vi "Get visa 1d DBL data.vi"(7 "VISA resource name":refnum<visa-resource-name>, 8 "error in (no error)":errorcluster, 9 "Name":string, 10 "Mag Lab Parameters in":refnum<class "Mag Lab Parameters.lvclass">, 11 "HP counter in":refnum<class "HP counter.lvclass">) -> (0 "error out":errorcluster, 1 "Channel data":dbl[](array[numeric]), 2 "Channel names":string[](array[string]), 3 "HP counter out":refnum<class "HP counter.lvclass">, 5 "VISA resource name out":refnum<visa-resource-name>)   [LabVIEW 2015, in "HP counter.lvclass"]
uses:
  HP counter.lvclass
  Mag Lab Properties/Mag Lab Parameters.lvclass
  Counter/Counter Parameters.ctl
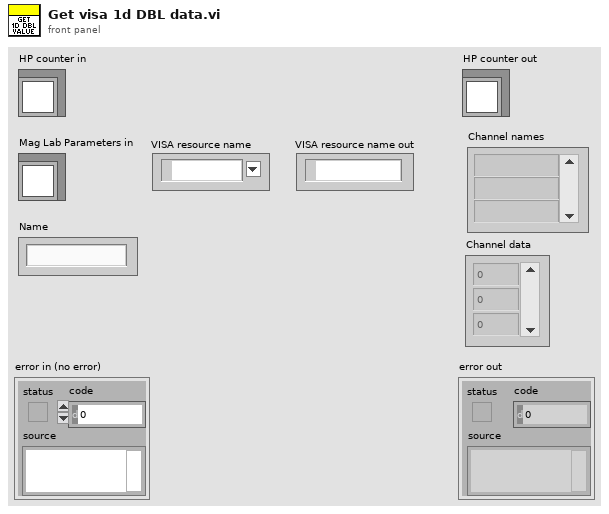
[diagram p1: front panel]
types:
  T1 = typedef "Counter Parameters.ctl" = cluster{"Channels to measure":i32[]}
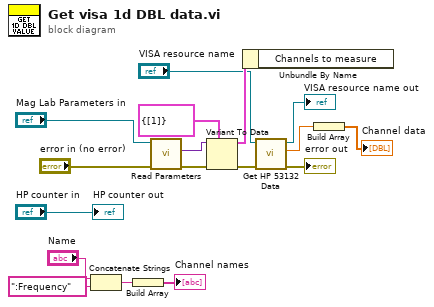
[diagram p0: block diagram]
diagram:
  n1 = Concatenate Strings("Name", ":Frequency" ("string")) -> (w7:string)
  n2 = Build Array(w7) -> (→"Channel names":string[])
  n3 = call-dynamic "Read Parameters.vi"("error in (no error)"="error in (no error)", "Mag Lab Parameters in"="Mag Lab Parameters in") -> ("error out"=w13:errorcluster, "Parameters"=w16:variant)  [unwired: 7 in, 1 out]
  n4 = Variant To Data(error in=w13, type=T1 {"Channels to measure"=[1]} ("Parameters"), Variant=w16) -> (data=w12:T1, error out=w11:errorcluster)
  n5 = Unbundle By Name(w12) -> ()  [unwired: 1 out]
  n6 = call "Get HP 53132 Data.vi"("error in (no error)"=w11, "VISA Resource Name"="VISA resource name") -> ("error out"=→"error out":errorcluster, "Data"=w3:dbl, "VISA Resource Name Out"=→"VISA resource name out":refnum<visa-resource-name>)  [unwired: 6 in]
  n7 = Build Array(w3) -> (→"Channel data":dbl[])
  "HP counter out" <- "HP counter in"
